vi "Test Style.vi"() -> ()   [LabVIEW 2020, in "ConstantErrorsMaker.lvlib"]
uses:
  ConstantErrorsMaker.lvlib
  MulticolumListbox.ctl
  <vilib>/National Instruments/Tree Map/API/List Roots.vi
  <vilib>/National Instruments/Tree Map/Utility/Into Tree Control Items.vi
  <vilib>/National Instruments/Tree Map/Tree Map.lvlib
panel:
  out "String Out":string
  in  "Button":bool
  in  "String":string="test text"
  in  "Tree Control":string(tree)
  in  "Boolean 2":bool
  in  "Blank Button":bool
  in  "OK Button":bool
  in  "Boolean":bool
  in  "Button 2":bool
  in  "Tank":dbl(slide) scale=0.0..10.0
  out "Numeric 2":dbl
  in  "Numeric":dbl
  in  "Multicolumn Listbox":T1
  in  "Results Listbox":T1
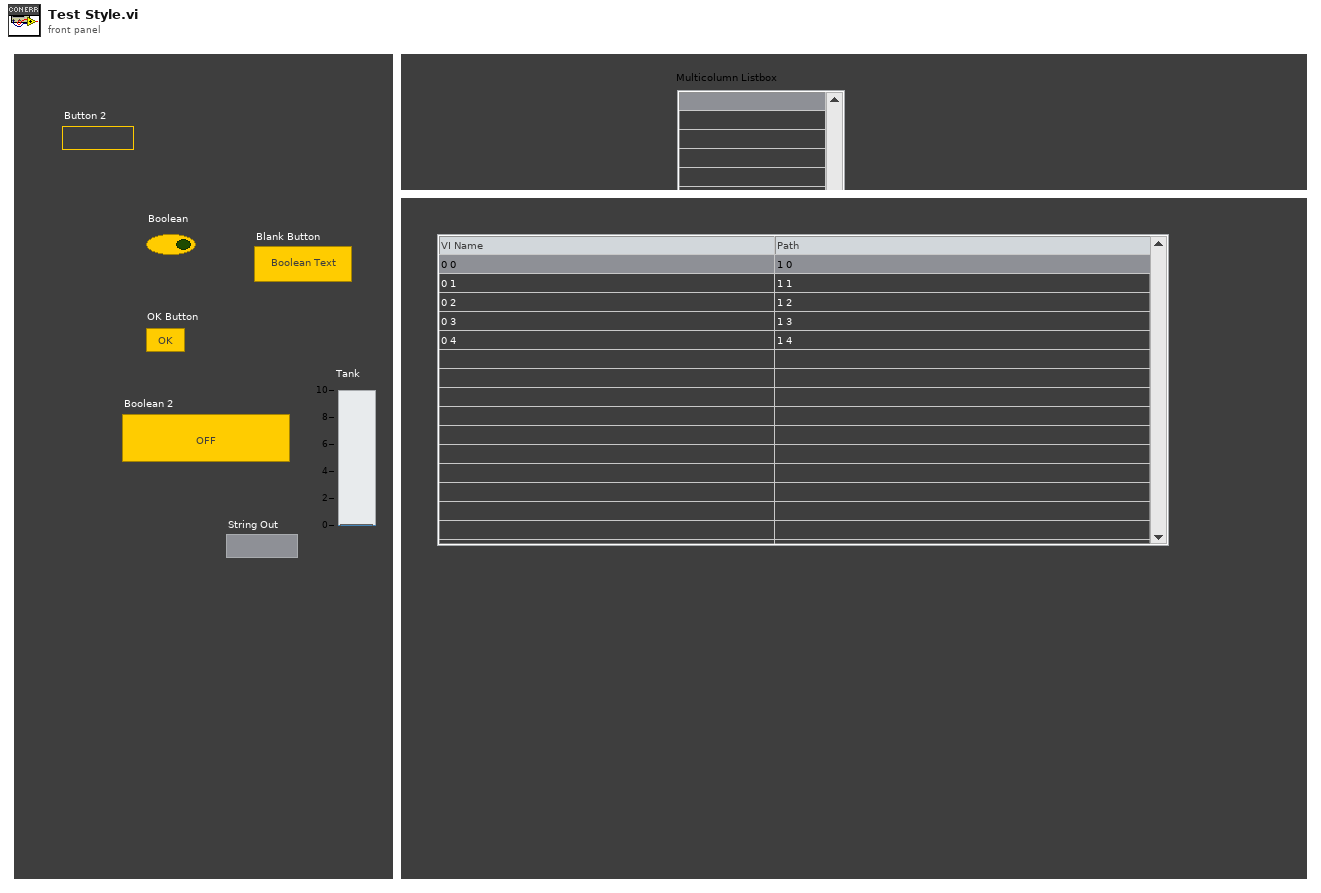
[diagram p1: front panel]
types:
  T1 = typedef "ConstantErrorsMaker.lvlib/MulticolumListbox.ctl" = i32
  T2 = typedef "Tree Map.lvlib/Tree Map Data.ctl" = map{string, cluster{"Child Paths Set":set{string}, "Name":string, "Data":string, "Attributes":map{string, string}}}
  T3 = cluster{"Left Cell String":string, "Child Text":string[], "Child Tag":string, "Item Indent":i32, "Child Only?":bool, "Glyph Index":i32}[]
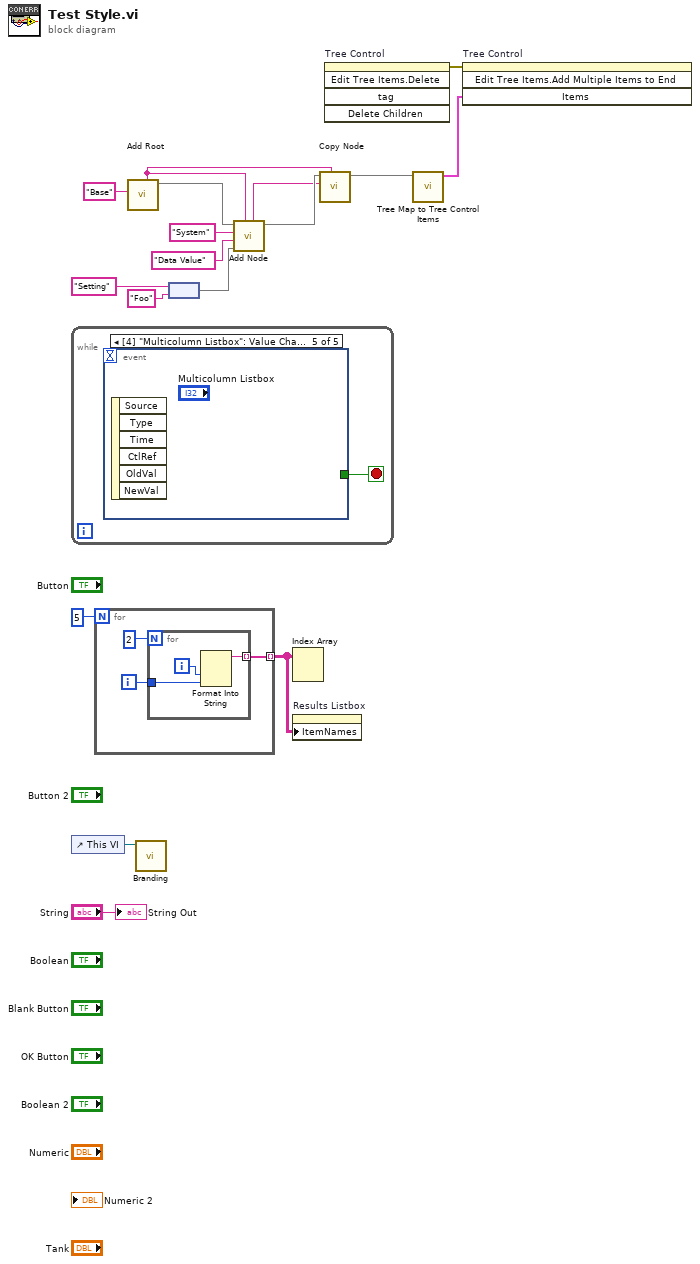
[diagram p0: block diagram]
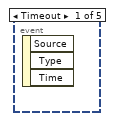
[diagram p2: hidden frame]
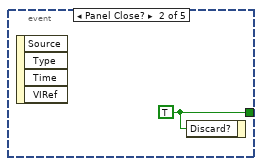
[diagram p3: hidden frame]
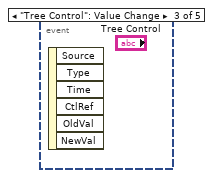
[diagram p4: hidden frame]
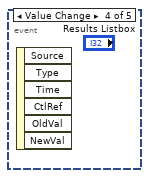
[diagram p5: hidden frame]
diagram:
  n1 = while {
    stop <- w18 stop-if-true
    n2 = event shown="[4] \"Multicolumn Listbox\": Value Change" {
      selector: _ -> [_ _ _ _ _]
      dyn-events: _ -> [_ _ _ _ _]
      timeout: _ -> [_ _ _ _ _]
      tunnel: [_ w19 _ _ _] -> w18
      event Timeout {
        n3 = event-data() -> ()  [unwired: 1 in, 3 out]
      }
      event Panel Close? {
        w19 = TRUE ("Discard?")
        n4 = event-data() -> ()  [unwired: 1 in, 4 out]
        n5 = event-data("Discard?"=w19) -> ()  [unwired: 1 in, 1 out]
      }
      event "Tree Control": Value Change {
        n6 = event-data() -> ()  [unwired: 1 in, 6 out]
      }
      event Value Change {
        n7 = event-data() -> ()  [unwired: 1 in, 6 out]
      }
      event Value Change {
        n8 = event-data() -> ()  [unwired: 1 in, 6 out]
      }
    }
  }
  n9 = control-ref of="This VI"() -> (w15:refnum<vi>)
  n10 = for {
    N: 5 -> [_]
    tunnel: [w21] -> w1 mode=indexing
    i -> [w22]
    n11 = for {
      N: 2 -> [_]
      tunnel: w22 -> [w24]
      tunnel: [w23] -> w21 mode=indexing
      i -> [w25]
      n12 = Format Into String(w25, w24) -> (resulting string=w23:string)  [unwired: 3 in, 1 out]
    }
  }
  n13 = call <vilib>:"Add Root.vi"("New Root Name"="Base") -> ("Tree Map Out"=w13:T2, "Root Path"=w5:string)  [unwired: 9 in]
  n14 = call "Branding.vi"("This VI"=w15) -> ()  [unwired: 11 in]
  n15 = node("Setting" ("New Root Name"), "Foo" ("New Root Name")) -> (w10:map{string, string})
  n16 = call <vilib>:"Add Node.vi"("Parent Path"=w5, "Attributes"=w10, "Data"="Data Value" ("New Root Name"), "New Node Name"="System" ("New Root Name"), "Tree Map In"=w13) -> ("Tree Map Out"=w4:T2, "New Node Path"=w3:string)  [unwired: 4 in, 1 out]
  n17 = Index Array(array=w1) -> ()  [unwired: 2 in, 1 out]
  n18 = property on="Results Listbox" class="MCListbox (strict)"("ItemNames"=w1) -> ()  [unwired: 2 in, 2 out]
  n19 = call <vilib>:"Copy Node.vi"("New Parent Path in Target"=w5, "Node Path in Source"=w3, "Target Tree Map In"=w4) -> ("Target Tree Map Out"=w6:T2)  [unwired: 6 in, 2 out]
  n20 = invoke on="Tree Control" class="Tree (strict)" method="Edit Tree Items.Delete"() -> (error out=w17:errorcluster)  [unwired: 5 in, 4 out]
  n21 = call <vilib>:"Tree Map to Tree Control Items.vi"("Tree Map In"=w6) -> ("Tree Control Items"=w7:T3)  [unwired: 10 in]
  n22 = invoke on="Tree Control" class="Tree (strict)" method="Edit Tree Items.Add Multiple Items to End"(error in=w17, "Items"=w7) -> ()  [unwired: 2 in, 4 out]
  "String Out" <- "String"
